vi "GetFlashJobFileList.vi"(8 "error in (no error)":errorcluster, 11 "SM1000-control in":T1) -> (0 "error out":errorcluster, 1 "Job list":string[](array[string]), 3 "SM1000-control out":T1)   [LabVIEW 2013, in "MaterialCharacterization.lvlib" / "MC-SM1000.lvclass"]
doc: "Returns a list of job files located on the Flash file system located on the EC1000.\n\nJobs are loaded into the EC1000 Flash file system through the use of the 'ILecSession.saveJobData' method.\n\nCommand: <\"GetFlashJobFileList\"> or 203\nReturns: array of stringss"
uses:
  MC-SM1000.lvclass
  Object-reference.ctl
  MC-SM1000.lvclass/MC-SM1000.ctl
  Custom-errors.ctl
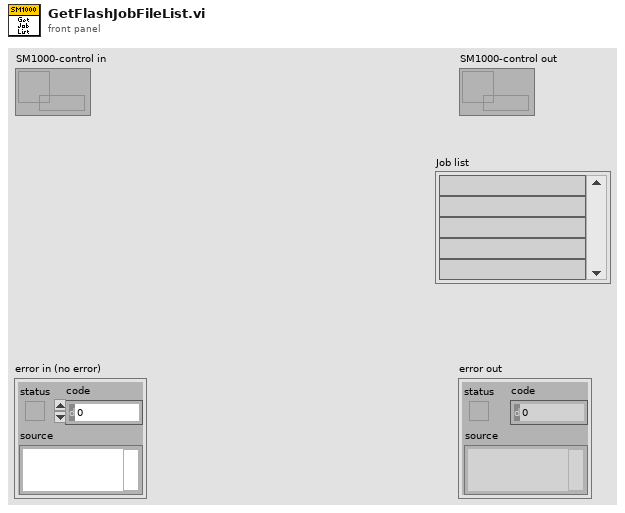
[diagram p1: front panel]
types:
  T1 = typedef "MaterialCharacterization.lvlib/MC-SM1000.lvclass/Object-reference.ctl" = refnum<data-value>
  T2 = typedef "MaterialCharacterization.lvlib/MC-SM1000.lvclass/Custom-errors.ctl" = enum16{"No error", "Not implemented", "Command not recognized", "Invalid input", "No connection", "Timeout", "Resource not loaded"}
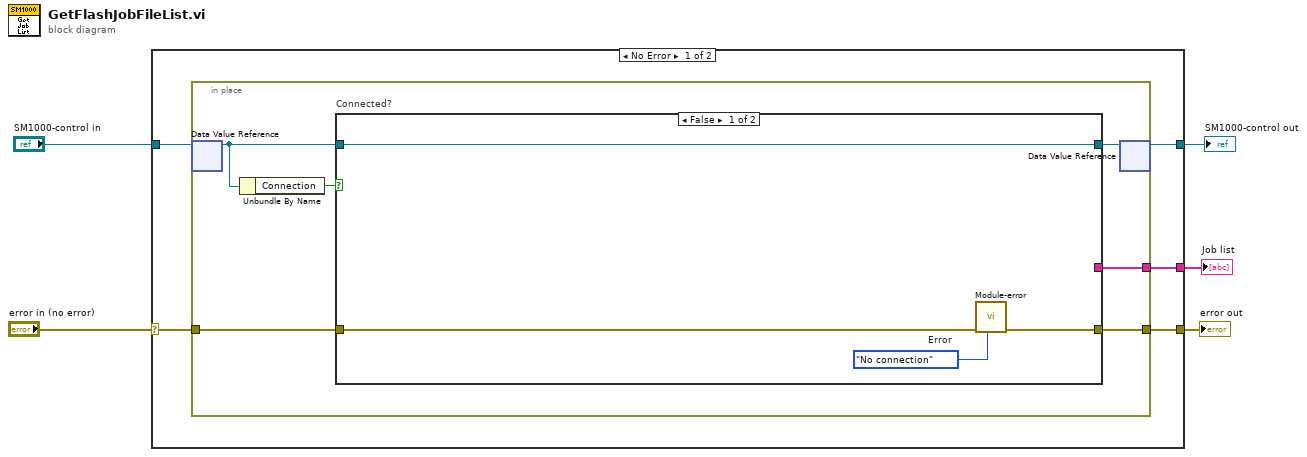
[diagram p0: block diagram]
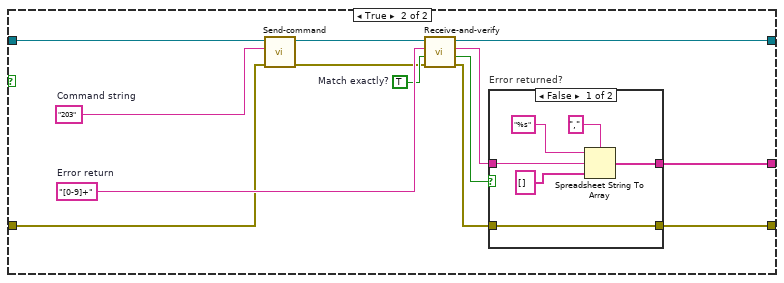
[diagram p2: hidden frame]
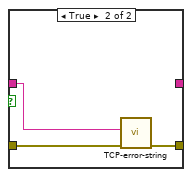
[diagram p3: hidden frame]
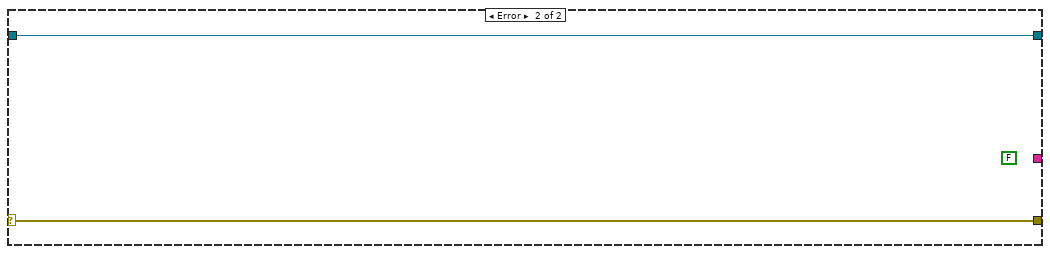
[diagram p4: hidden frame]
diagram:
  n1 = case shown="No Error" "error in (no error)" {
    selector: "error in (no error)" -> [w8 w44]
    tunnel: [w7 w44] -> w4
    tunnel: [w9 w43] -> w2
    tunnel: "SM1000-control in" -> [w10 w43]
    tunnel: [w6 _] -> w1
    frame No Error {
      n2 = in-place {
        in-place-border: w8 -> [w16]
        in-place-border: [w13] -> w7
        in-place-border: [w11] -> w6
        n3 = in-place-dvr #1(w10) -> (w14:refnum<class "MC-SM1000.lvclass">)  [unwired: 1 out]
        n4 = Unbundle By Name(w14) -> ("Connection"=w15:bool)
        n5 = case "Connected?" shown="False" w15 {
          tunnel: w16 -> [w20 w26]
          tunnel: w14 -> [w18 w33]
          tunnel: [w19 w24] -> w13
          tunnel: [w18 w23] -> w12
          tunnel: [_ w22] -> w11
          frame False {
            w17 = Custom-errors."No connection"  # Error
            n6 = call "Module-error.vi"("Error"=w17, "error in (no error)"=w20) -> ("error out"=w19:errorcluster)  [unwired: 9 in]
          }
          frame True {
            w30 = TRUE  # Match exactly?
            w31 = "[0-9]+"  # Error return
            w21 = "203"  # Command string
            n7 = call "Send-command.vi"("error in (no error)"=w26, "Command string"=w21, "SM1000-control in"=w33) -> ("error out"=w29:errorcluster, "SM1000-control out"=w32:refnum<class "MC-SM1000.lvclass">)  [unwired: 7 in]
            n8 = call "Receive-and-verify.vi"("error in (no error)"=w29, "Match exactly?"=w30, "Expected return string"=w31, "SM1000-control in"=w32) -> ("error out"=w25:errorcluster, "Verified?"=w28:bool, "Return string"=w27:string, "SM1000-control out"=w23:refnum<class "MC-SM1000.lvclass">)  [unwired: 4 in]
            n9 = case "Error returned?" shown="False" w28 {
              tunnel: w27 -> [w38 w40]
              tunnel: w25 -> [w39 w41]
              tunnel: [w39 w42] -> w24
              tunnel: [w35 _] -> w22
              frame False {
                n10 = Spreadsheet String To Array(delimiter (Tab)=",", format string="%s", spreadsheet string=w38, array type (2D Dbl)=string[] []) -> (array=w35:string[])
              }
              frame True {
                n11 = call "TCP-error-string.vi"("error in (no error)"=w41, "Retun code"=w40) -> ("error out"=w42:errorcluster)  [unwired: 9 in]
              }
            }
          }
        }
        n12 = in-place-dvr #1(w12) -> (w9:T1)  [unwired: 1 out]
      }
    }
    frame Error {
      (unwired) FALSE
    }
  }
  "error out" <- w4
  "SM1000-control out" <- w2
  "Job list" <- w1
